vi "Curcular Buffer Data History.vi"(6 "Oldest time to Plot":dbl, 7 "write (F)":bool, 8 "Error In":errorcluster, 9 "Data Value":dbl, 10 "Time Stamp":dbl format="%^<%H:%M:%S%4u\n%x>T", 11 "Device Name":string) -> (0 "Error Out":errorcluster, 1 "Latest Timestamp":dbl, 2 "Latest Value":dbl, 3 "Truncated Data History":T1)   [LabVIEW 2015]
uses:
  typedefs/DVR Map Action.ctl
  typedefs/Data History.ctl
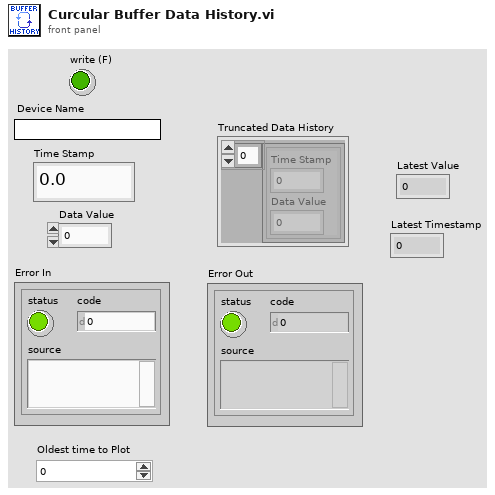
[diagram p1: front panel]
types:
  T1 = cluster{cluster{"Time Stamp":dbl, "Data Value":dbl}[]}
  T2 = typedef "DVR Map Action.ctl" = enum16{"Read Names", "Write", "Read"}
  T3 = typedef "Data History.ctl" = cluster{"Timestamps":dbl[], "Values":dbl[]}
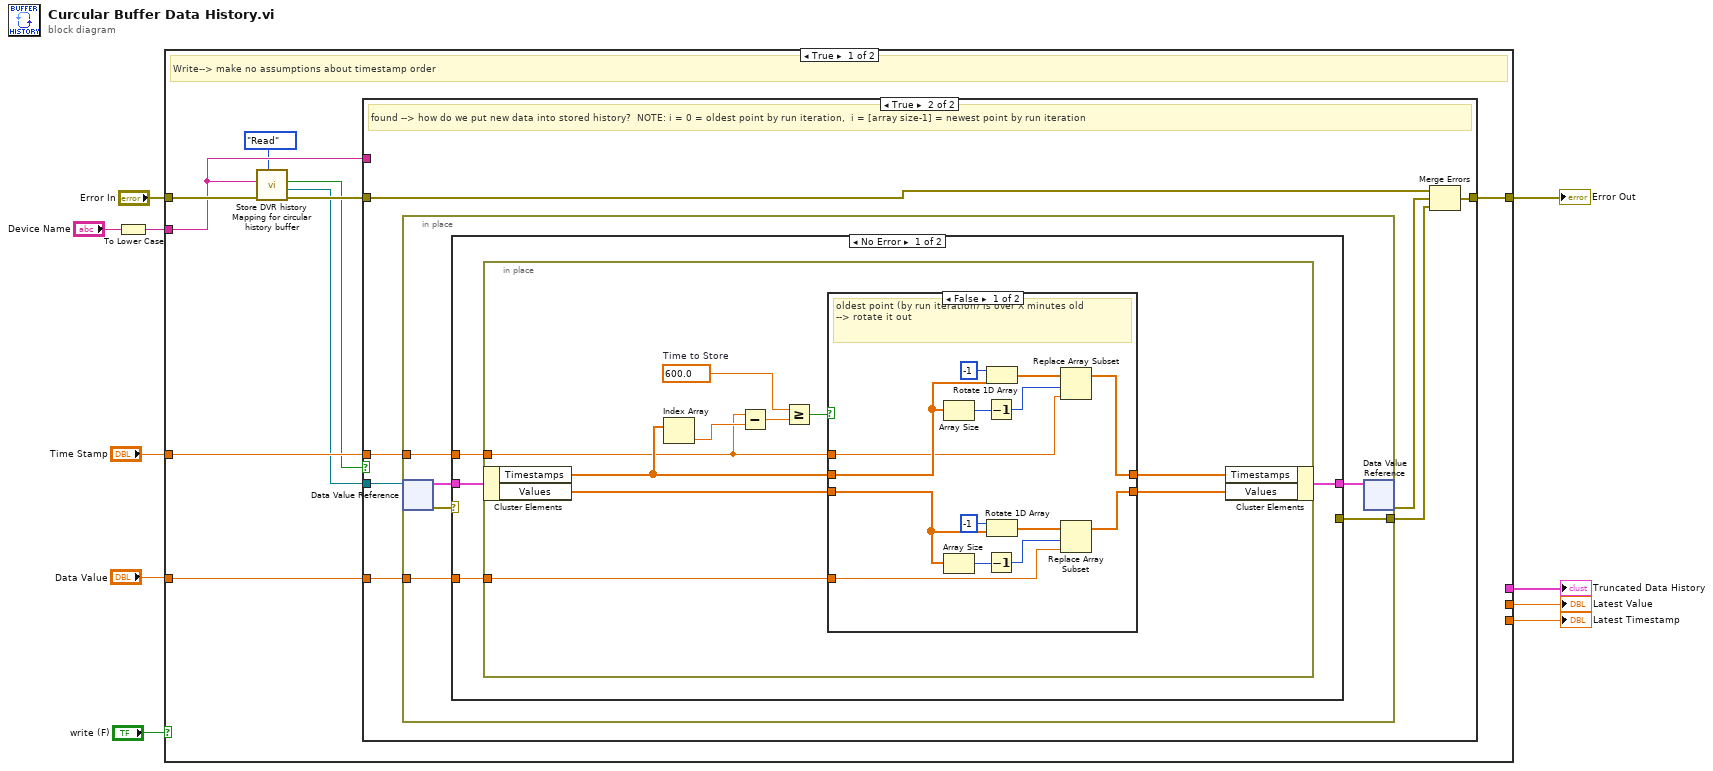
[diagram p0: block diagram]
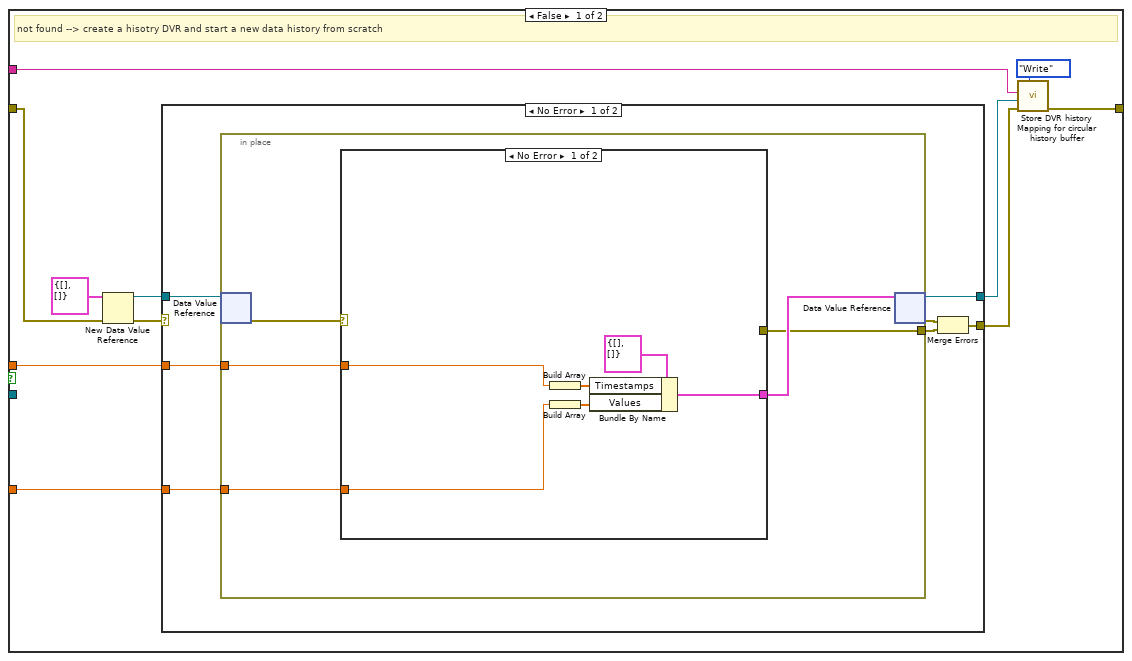
[diagram p2: hidden frame]
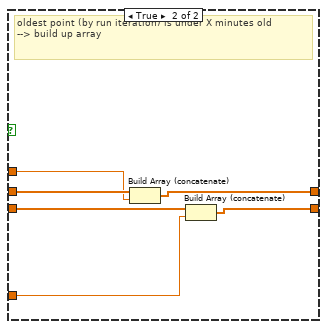
[diagram p5: hidden frame]
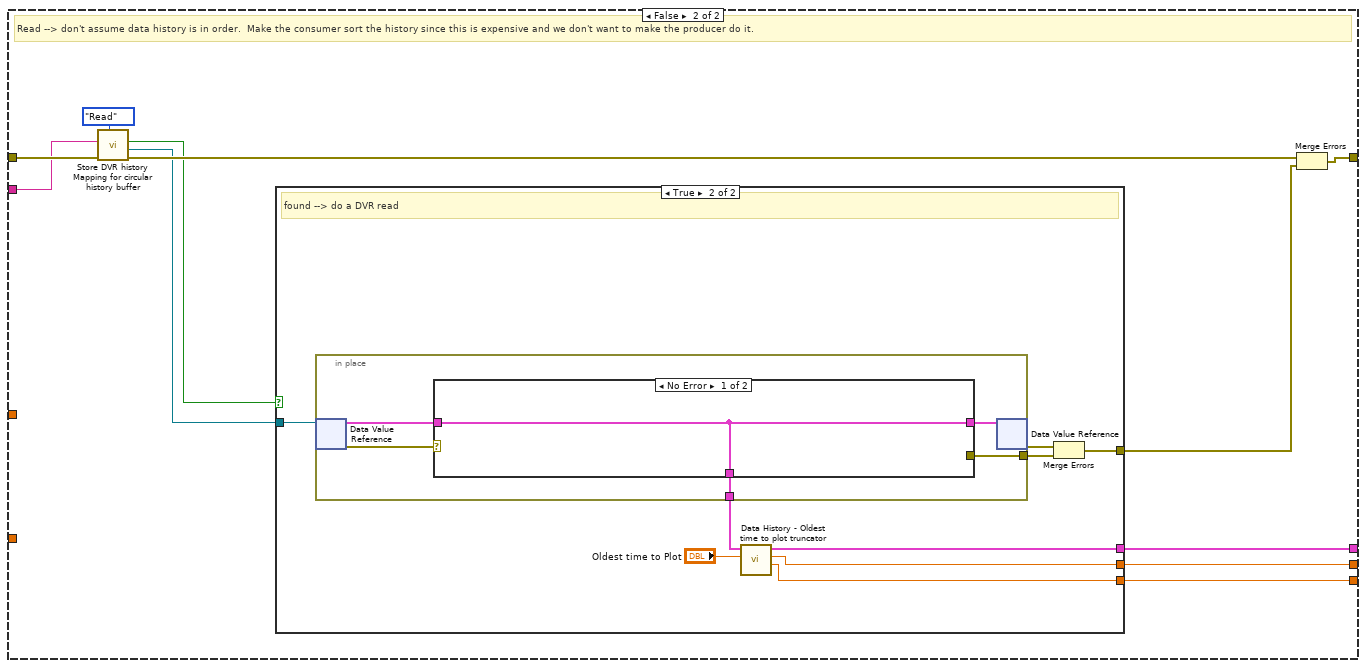
[diagram p7: hidden frame]
diagram:
  n1 = To Lower Case(string="Device Name") -> (all lower case string=w2:string)
  n2 = case shown="True" "write (F)" {
    tunnel: w2 -> [w12 w100]
    tunnel: "Time Stamp" -> [w19 _]
    tunnel: "Data Value" -> [w18 _]
    tunnel: [w17 w108] -> w6
    tunnel: "Error In" -> [w16 w104]
    tunnel: [_ w107] -> w3
    tunnel: [_ w106] -> w5
    tunnel: [_ w105] -> w4
    frame True {
      # "Write--> make no assumptions about timestamp order"
      n3 = call "Store DVR history Mapping for circular history buffer.vi"("Action"=DVR_Map_Action."Read", "error in"=w16, "Device Name"=w12) -> ("error out"=w15:errorcluster, "History DVR"=w13:refnum<data-value>, "Found?"=w14:bool)  [unwired: 5 in, 1 out]
      n4 = case shown="True" w14 {
        tunnel: w13 -> [_ w55]
        tunnel: w19 -> [w30 w57]
        tunnel: w18 -> [w29 w56]
        tunnel: w12 -> [w21 _]
        tunnel: w15 -> [w26 w51]
        tunnel: [w23 w54] -> w17
        frame False {
          # "not found --> create a hisotry DVR and start a new data history from scratch"
          n5 = New Data Value Reference(data value=T3 {"Timestamps"=[], "Values"=[]} ("Current Value Data"), error in=w26) -> (data value reference=w27:refnum<data-value>, error out=w25:errorcluster)
          n6 = case shown="No Error" w25 {
            selector: w25 -> [_ w50]
            tunnel: w30 -> [w37 _]
            tunnel: w29 -> [w36 _]
            tunnel: w27 -> [w35 _]
            tunnel: [w32 w50] -> w24
            tunnel: [w31 _] -> w22
            frame No Error {
              n7 = in-place {
                in-place-border: w37 -> [w42]
                in-place-border: w36 -> [w41]
                in-place-border: [w38] -> w33
                n8 = in-place-dvr #1(w35) -> (w40:errorcluster)  [unwired: 1 out]
                n9 = case shown="No Error" w40 {
                  selector: w40 -> [_ w49]
                  tunnel: w42 -> [w47 _]
                  tunnel: w41 -> [w46 _]
                  tunnel: [w43 _] -> w39
                  tunnel: [_ w49] -> w38
                  frame No Error {
                    n10 = Build Array(w47) -> (w45:dbl[])
                    n11 = Build Array(w46) -> (w44:dbl[])
                    n12 = Bundle By Name(cluster=T3 {"Timestamps"=[], "Values"=[]} ("Current Value Data"), "Timestamps"=w45, "Values"=w44) -> (w43:T3)
                  }
                  frame Error {
                  }
                }
                n13 = in-place-dvr #1(w39) -> (w31:refnum<data-value>, w34:errorcluster)
              }
              n14 = Merge Errors(w34, w33) -> (w32:errorcluster)
            }
            frame Error {
            }
          }
          n15 = call "Store DVR history Mapping for circular history buffer.vi"("Action"=DVR_Map_Action."Write", "error in"=w24, "History DVR"=w22, "Device Name"=w21) -> ("error out"=w23:errorcluster)  [unwired: 4 in, 3 out]
        }
        frame True {
          # "found --> how do we put new data into stored history?  NOTE: i = 0 = oldest point by run iteration,  i = [array size-1] = newest point by run iteration"
          n16 = in-place {
            in-place-border: w57 -> [w62]
            in-place-border: w56 -> [w63]
            in-place-border: [w58] -> w53
            n17 = in-place-dvr #2(w55) -> (w60:T3, w61:errorcluster)
            n18 = case shown="No Error" w61 {
              selector: w61 -> [_ w98]
              tunnel: w63 -> [w67 _]
              tunnel: w62 -> [w66 _]
              tunnel: w60 -> [w65 _]
              tunnel: [w64 _] -> w59
              tunnel: [_ w98] -> w58
              frame No Error {
                n19 = in-place {
                  in-place-border: w67 -> [w77]
                  in-place-border: w66 -> [w68]
                  w72 = 600.0  # Time to Store
                  n20 = in-place-cluster #3(w65) -> ("Timestamps"=w76:dbl[], "Values"=w75:dbl[])
                  n21 = Index Array(array=w76) -> (element=w71:dbl)  [unwired: 1 in]
                  n22 = Subtract(x=w68, y=w71) -> (x-y=w70:dbl)
                  n23 = Greater Or Equal?(x=w72, y=w70) -> (x >= y?=w69:bool)
                  n24 = case shown="False" w69 {
                    tunnel: w75 -> [w83 w94]
                    tunnel: w77 -> [w82 w93]
                    tunnel: [w81 w95] -> w74
                    tunnel: [w80 w92] -> w73
                    tunnel: w76 -> [w79 w97]
                    tunnel: w68 -> [w78 w96]
                    frame False {
                      # "oldest point (by run iteration) is over X minutes old\n--> rotate it out"
                      n25 = Array Size(array=w79) -> (size(s)=w88:i32)
                      n26 = Array Size(array=w83) -> (size(s)=w87:i32)
                      n27 = Decrement(x=w88) -> (x-1=w91:i32)
                      n28 = Decrement(x=w87) -> (x-1=w84:i32)
                      n29 = Rotate 1D Array(1:w79, 2:-1 ("n")) -> (0:w90:dbl[])
                      n30 = Rotate 1D Array(1:w83, 2:-1 ("n")) -> (0:w85:dbl[])
                      n31 = Replace Array Subset(array=w90, new element=w78, index=w91) -> (w81:dbl[])
                      n32 = Replace Array Subset(array=w85, new element=w82, index=w84) -> (w80:dbl[])
                    }
                    frame True {
                      # "oldest point (by run iteration) is under X minutes old\n--> build up array"
                      n33 = Build Array (concatenate)(w97, w96) -> (w95:dbl[])
                      n34 = Build Array (concatenate)(w94, w93) -> (w92:dbl[])
                    }
                  }
                  n35 = in-place-cluster #3("Timestamps"=w74, "Values"=w73) -> (w64:T3)
                }
              }
              frame Error {
              }
            }
            n36 = in-place-dvr #2(w59) -> (w52:errorcluster)  [unwired: 1 out]
          }
          n37 = Merge Errors(w51, w52, w53) -> (w54:errorcluster)
        }
      }
    }
    frame False {
      # "Read --> don't assume data history is in order.  Make the consumer sort the history since this is expensive and we don't want to make the producer do it."
      n38 = call "Store DVR history Mapping for circular history buffer.vi"("Action"=DVR_Map_Action."Read", "error in"=w104, "Device Name"=w100) -> ("error out"=w103:errorcluster, "History DVR"=w102:refnum<data-value>, "Found?"=w101:bool)  [unwired: 5 in, 1 out]
      n39 = case shown="True" w101 {
        tunnel: w102 -> [_ w118]
        tunnel: [_ w115] -> w109
        tunnel: [_ w113] -> w107
        tunnel: [_ w111] -> w106
        tunnel: [_ w112] -> w105
        frame False {
          # "not found --> return empty data"
        }
        frame True {
          # "found --> do a DVR read"
          n40 = in-place {
            in-place-border: [w120] -> w116
            in-place-border: [w119] -> w110
            n41 = in-place-dvr #4(w118) -> (w122:T3, w123:errorcluster)
            n42 = case shown="No Error" w123 {
              selector: w123 -> [_ w125]
              tunnel: w122 -> [w124 w126]
              tunnel: [w124 w126] -> w121
              tunnel: [_ w125] -> w120
              tunnel: [w124 _] -> w119
              frame No Error {
              }
              frame Error {
              }
            }
            n43 = in-place-dvr #4(w121) -> (w117:errorcluster)  [unwired: 1 out]
          }
          n44 = call "Data History - Oldest time to plot truncator.vi"("Oldest Time To Plot"="Oldest time to Plot", "Full History Data"=w110) -> ("Latest Timestamp"=w112:dbl, "Latest Value"=w111:dbl, "Truncated Data History"=w113:T1)  [unwired: 7 in]
          n45 = Merge Errors(w117, w116) -> (w115:errorcluster)
        }
      }
      n46 = Merge Errors(w103, w109) -> (w108:errorcluster)
    }
  }
  "Error Out" <- w6
  "Latest Value" <- w5
  "Latest Timestamp" <- w4
  "Truncated Data History" <- w3
